vi "UserName.vi"(8 "error in (no error)":errorcluster, 11 "FTP in":refnum<class "FTP.lvclass">) -> (0 "error out":errorcluster, 3 "FTP out":refnum<class "FTP.lvclass">)   [LabVIEW 2017, in "FTP_UpgradeCSMF.lvlib" / "FTP.lvclass"]
uses:
  FTP.lvclass
  FTP.lvclass/FTP.ctl
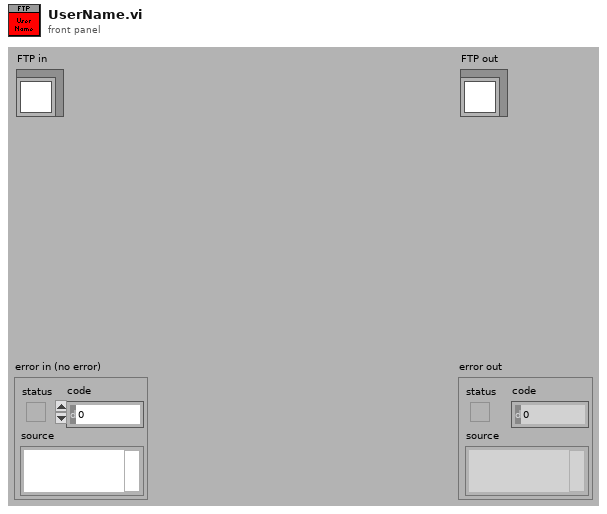
[diagram p1: front panel]
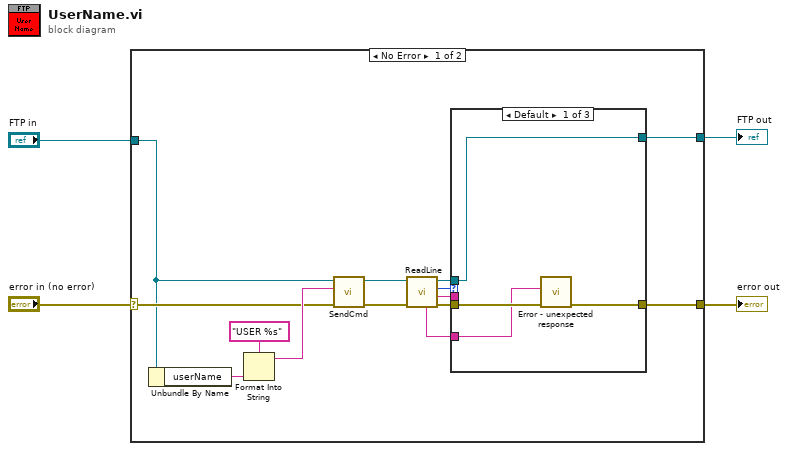
[diagram p0: block diagram]
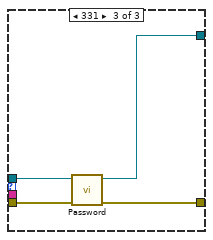
[diagram p3: hidden frame]
diagram:
  n1 = case shown="No Error" "error in (no error)" {
    selector: "error in (no error)" -> [w14 w30]
    tunnel: [w12 w30] -> w3
    tunnel: [w13 w29] -> w1
    tunnel: "FTP in" -> [w11 w29]
    frame No Error {
      n2 = Unbundle By Name(w11) -> ("userName"=w10:string)
      n3 = Format Into String(format string="USER %s", w10) -> (resulting string=w16:string)  [unwired: 2 in, 1 out]
      n4 = call "SendCmd.vi"("error in (no error)"=w14, "cmd"=w16, "FTP in"=w11) -> ("error out"=w17:errorcluster, "FTP out"=w18:refnum<class "FTP.lvclass">)  [unwired: 7 in]
      n5 = call "ReadLine.vi"("error in (no error)"=w17, "FTP in"=w18) -> ("error out"=w9:errorcluster, "Line"=w6:string, "code"=w8:i32, "FTP out"=w7:refnum<class "FTP.lvclass">, "Full Line"=w5:string)  [unwired: 5 in]
      n6 = case shown="Default" w8 {
        tunnel: w9 -> [w21 w23 w28]
        tunnel: w7 -> [w22 w24 w27]
        tunnel: [w22 w24 w25] -> w13
        tunnel: [w20 w23 w26] -> w12
        tunnel: w6 -> [_ _ _]
        tunnel: w5 -> [w19 _ _]
        frame Default {
          n7 = call "Error - unexpected response.vi"("error in (no error)"=w21, "Full Response"=w19) -> ("error out"=w20:errorcluster)  [unwired: 9 in]
        }
        frame 200..299 {
        }
        frame 331 {
          n8 = call "Password.vi"("error in (no error)"=w28, "FTP in"=w27) -> ("error out"=w26:errorcluster, "FTP out"=w25:refnum<class "FTP.lvclass">)  [unwired: 8 in]
        }
      }
    }
    frame Error {
    }
  }
  "error out" <- w3
  "FTP out" <- w1
